vi "Humid Air 3BC & Mass Flow Rate of Dry Air To Mass Flow Rate of Humid Air.vi"(1 "Gas Presure":dbl[unit]=80000.0 min=80000.0 max=120000.0, 2 "Tceg":dbl[unit], 3 "M dot_DA":dbl[unit], 4 "RH":dbl) -> (0 "Mdot_HA":dbl[unit])   [LabVIEW 2018]
panel:
  out "Humidity of Input Air":dbl(knob) scale=0.0..100.0
  out "Temprature Of Input Air\nKelvin Degree":dbl[unit](slide) scale=273.0..373.0
  out "Tk":dbl[unit]
  out "Temprature Of Input Air\nCentigrade Degree":dbl[unit](slide) scale=0.0..100.0
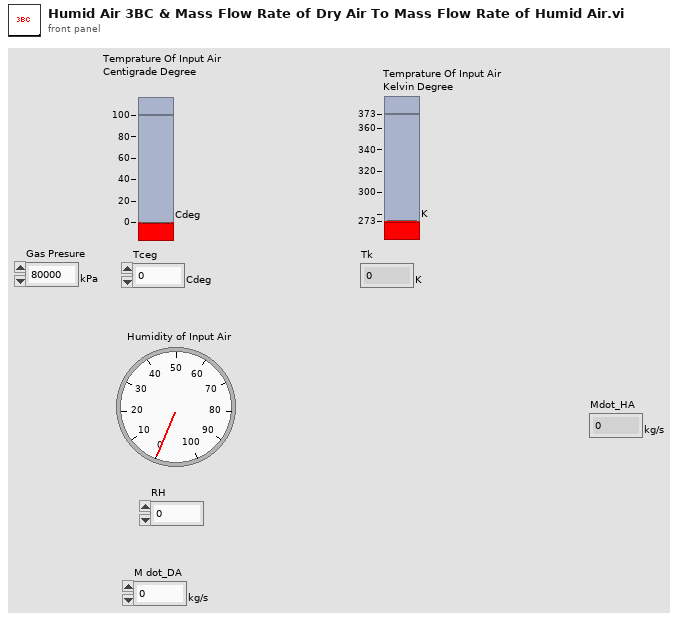
[diagram p1: front panel]
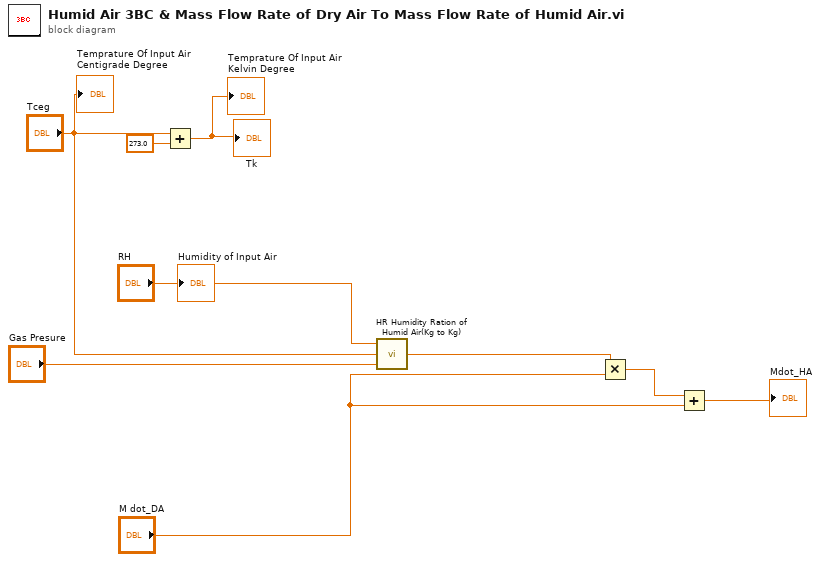
[diagram p0: block diagram]
diagram:
  n1 = Add(x="Tceg", y=dbl[unit] 273.0) -> (x+y=→"Tk" →"Temprature Of Input Air\nKelvin Degree":dbl[unit])
  n2 = call "HR Humidity Ration of Humid Air(Kg to Kg).vi"("Gas Presure"="Gas Presure", "Tceg"="Tceg", "RH"="RH") -> ("HR"=w4:dbl)
  n3 = Multiply(x=w4, y="M dot_DA") -> (x*y=w7:dbl[unit])
  n4 = Add(x=w7, y="M dot_DA") -> (x+y=→"Mdot_HA":dbl[unit])
  "Temprature Of Input Air\nCentigrade Degree" <- "Tceg"
  "Humidity of Input Air" <- "RH"
